vi "GetRevInfo.vi"(0 "MLA":refnum<class "MLA.lvclass">, 5 "error in (no error)":errorcluster) -> (14 "MLA":refnum<class "MLA.lvclass">, 15 "Test Software PN":string, 16 "Test Software Version":string, 17 "S5 Version":string, 18 "Revision History":string, 19 "error out":errorcluster)   [LabVIEW 2023, in "MLA.lvclass"]
uses:
  MLA.lvclass
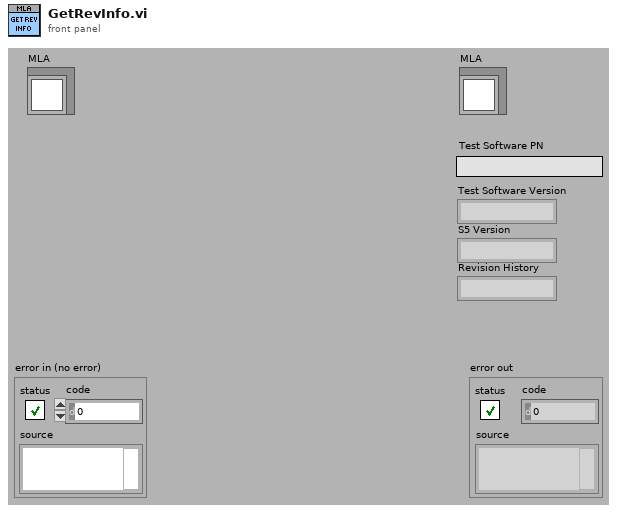
[diagram p1: front panel]
types:
  T1 = typedef "MLA.lvclass/ObjectAttributes.ctl" = cluster{"App Name":string, "App Version":string, "Revision History":string, "Log File Path":path, "Config INI File":path, "Config Path":path, "Log Archive Path":path, "Msg Q's":refnum<queue>[], "VI":refnum<vi>, "ErrLog":refnum<class "ErrorLog.lvclass">}
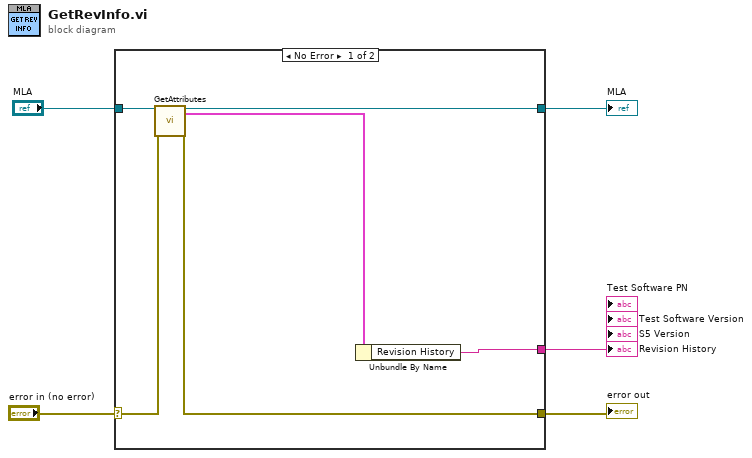
[diagram p0: block diagram]
diagram:
  n1 = case shown="No Error" "error in (no error)" {
    selector: "error in (no error)" -> [w11 w13]
    tunnel: [w9 w13] -> w4
    tunnel: [w7 w12] -> w2
    tunnel: "MLA" -> [w8 w12]
    tunnel: [w6 _] -> w1
    frame No Error {
      n2 = call "GetAttributes.vi"("MLA"=w8, "error in (no error)"=w11) -> ("MLA"=w7:refnum<class "MLA.lvclass">, "Data"=w10:T1, "error out"=w9:errorcluster)  [unwired: 14 in, 1 out]
      n3 = Unbundle By Name(w10) -> ("Revision History"=w6:string)
    }
    frame Error {
    }
  }
  "error out" <- w4
  "MLA" <- w2
  "Revision History" <- w1
